vi "cluster10.vi"() -> ()   [LabVIEW 2021]
panel:
  out "Gauge 2":dbl(knob) scale=0.0..10.0
  out "Gauge":dbl(knob) scale=0.0..10.0
  in  "Knob 2":dbl(knob) scale=0.0..10.0
  in  "Knob":dbl(knob) scale=0.0..10.0
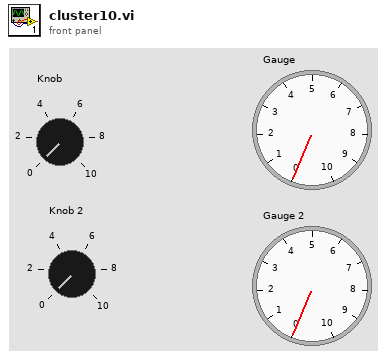
[diagram p1: front panel]
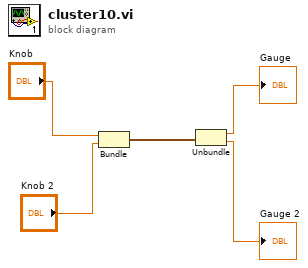
[diagram p0: block diagram]
diagram:
  n1 = Bundle("Knob"="Knob", "Knob 2"="Knob 2") -> (w3:cluster{"Knob":dbl, "Knob 2":dbl})  [unwired: 1 in]
  n2 = Unbundle(w3) -> ("Knob"=→"Gauge":dbl, "Knob 2"=→"Gauge 2":dbl)
